vi "UWB_data_extractor.vi"(11 "Data":u8[](array[numeric])) -> (0 "quality":u8, 1 "Z value (mm)":i32, 2 "Y value (mm)":i32, 3 "X value (mm)":i32)   [LabVIEW 2016]
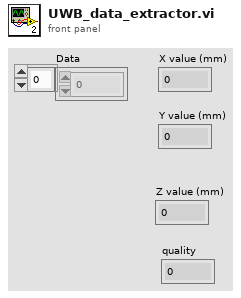
[diagram p1: front panel]
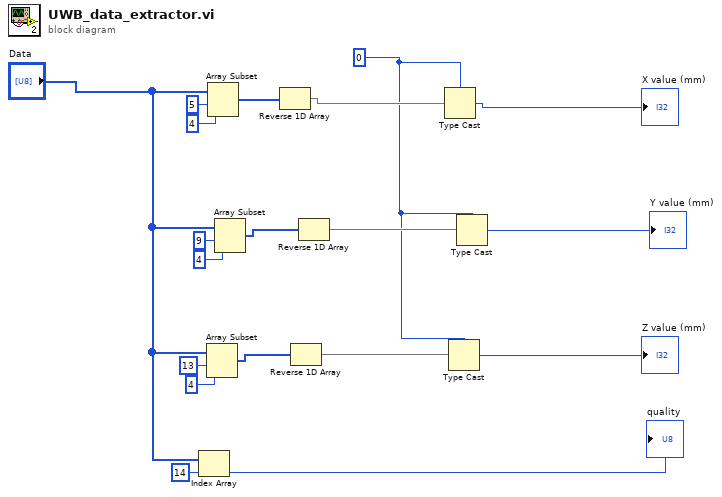
[diagram p0: block diagram]
diagram:
  w4 = 0
  n1 = Index Array(array="Data", index=14) -> (element=→"quality":u8)
  n2 = Array Subset(array="Data", index=13, length=4) -> (w6:u8[])
  n3 = Array Subset(array="Data", index=5, length=4) -> (w13:u8[])
  n4 = Array Subset(array="Data", index=9, length=4) -> (w11:u8[])
  n5 = Reverse 1D Array(array=w13) -> (reversed array=w12:u8[])
  n6 = Reverse 1D Array(array=w6) -> (reversed array=w5:u8[])
  n7 = Reverse 1D Array(array=w11) -> (reversed array=w10:u8[])
  n8 = Type Cast(type=w4, x=w12) -> (*(type *) &x=→"X value (mm)":i32)
  n9 = Type Cast(type=w4, x=w5) -> (*(type *) &x=→"Z value (mm)":i32)
  n10 = Type Cast(type=w4, x=w10) -> (*(type *) &x=→"Y value (mm)":i32)
